vi "CheckShot2Invader_new.vi"(6 "IntensityArray_IN":u8[][](array[numeric]), 7 "InvaderPosArray_IN":T1, 11 "ShotArray_IN":T3[](array[typedef])) -> (3 "ShotArray_OUT":T3[](array[typedef]), 4 "IntensityArray_OUT":u8[][](array[numeric]), 5 "InvaderPosArray_OUT":T1)   [LabVIEW 2022 SP3]
uses:
  InvaderPositionArray.ctl
  move_dir_lr.ctl
  ShotCluster.ctl
  move_dir_ud.ctl
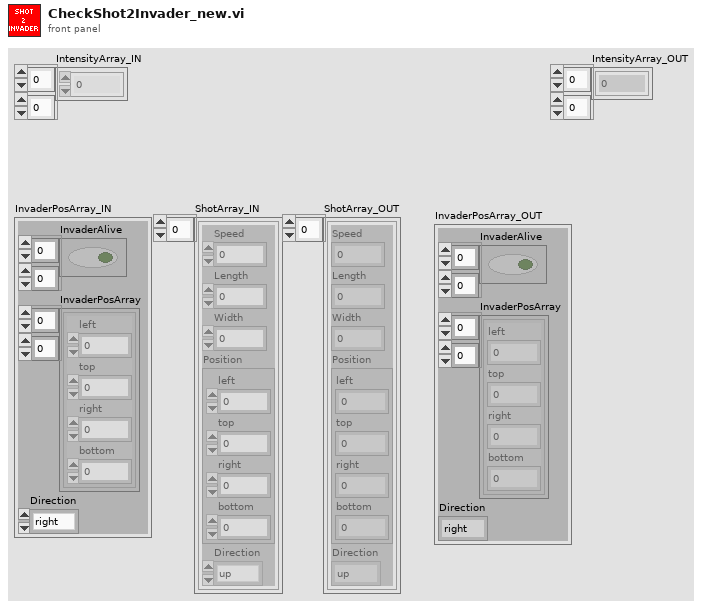
[diagram p1: front panel]
types:
  T1 = typedef "InvaderPositionArray.ctl" = cluster{"InvaderAlive":bool[][], "InvaderPosArray":cluster{"left":i16, "top":i16, "right":i16, "bottom":i16}[][], "Direction":T2}
  T2 = typedef "move_dir_lr.ctl" = enum16{"right", "left"}
  T3 = typedef "ShotCluster.ctl" = cluster{"Speed":u32, "Length":u32, "Width":u32, "Position":cluster{"left":i16, "top":i16, "right":i16, "bottom":i16}, "Direction":T4}
  T4 = typedef "move_dir_ud.ctl" = enum16{"up", "down"}
  T5 = cluster{"left":i16, "top":i16, "right":i16, "bottom":i16}[][]
  T6 = cluster{"left":i16, "top":i16, "right":i16, "bottom":i16}
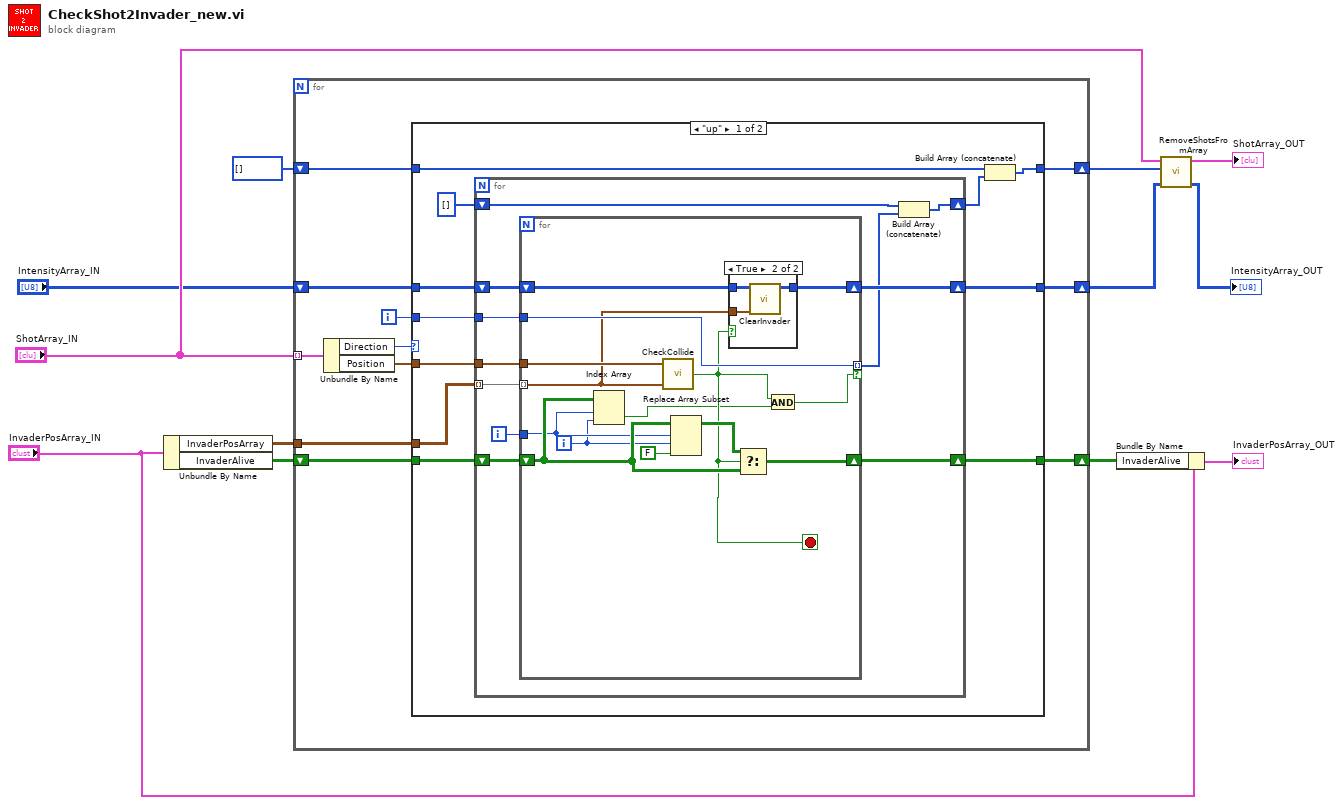
[diagram p0: block diagram]
diagram:
  n1 = Unbundle By Name("InvaderPosArray_IN") -> ("InvaderPosArray"=w1:T5, "InvaderAlive"=w12:bool[][])
  n2 = for {
    tunnel: "ShotArray_IN" -> [w23] mode=indexing
    shift-right: [w19] -> w11
    shift-left: w12 -> [w21]
    shift-right: [w16] -> w5
    shift-left: i32[] [] -> [w17]
    shift-right: [w14] -> w4
    shift-left: "IntensityArray_IN" -> [w15]
    tunnel: w1 -> [w13]
    i -> [w18]
    n3 = Unbundle By Name(w23) -> ("Direction"=w22:T4, "Position"=w20:T6)
    n4 = case shown="\"up\"" w22 {
      tunnel: w21 -> [w33 w66]
      tunnel: w20 -> [w34 _]
      tunnel: [w32 w66] -> w19
      tunnel: w18 -> [w31 _]
      tunnel: w17 -> [w30 w65]
      tunnel: [w28 w65] -> w16
      tunnel: w15 -> [w27 w64]
      tunnel: [w26 w64] -> w14
      tunnel: w13 -> [w25 _]
      frame "up" {
        n5 = for {
          tunnel: w34 -> [w45]
          tunnel: w31 -> [w42]
          tunnel: w25 -> [w39] mode=indexing
          shift-right: [w40] -> w26
          shift-left: w27 -> [w41]
          shift-right: [w38] -> w29
          shift-left: i32[] [] -> [w37]
          shift-right: [w43] -> w32
          shift-left: w33 -> [w44]
          i -> [w35]
          n6 = for {
            tunnel: w45 -> [w59]
            shift-right: [w58] -> w43
            shift-left: w44 -> [w51]
            tunnel: w42 -> [w57]
            tunnel: [w57] -> w36 mode=indexing if=w46
            shift-right: [w55] -> w40
            shift-left: w41 -> [w56]
            tunnel: w39 -> [w54] mode=indexing
            tunnel: w35 -> [w50]
            i -> [w49]
            stop <- w48 stop-if-true
            n7 = Index Array(array=w51, index (row)=w50, index (col)=w49) -> (element=w47:bool)
            n8 = call "CheckCollide.vi"("Rectangle2"=w54, "Rectangle1"=w59) -> ("Collide"=w48:bool)  [unwired: 3 in]
            n9 = Replace Array Subset(array=w51, new element=FALSE, index (row)=w50, index (col)=w49) -> (w52:bool[][])
            n10 = case shown="True" w48 {
              tunnel: w56 -> [w60 w63]
              tunnel: [w60 w62] -> w55
              tunnel: w54 -> [_ w61]
              frame False {
              }
              frame True {
                n11 = call "ClearInvader.vi"("InvaderPosition"=w61, "IntensityArray_IN"=w63) -> ("IntensityArray_OUT"=w62:u8[][])  [unwired: 9 in]
              }
            }
            n12 = Select(t=w52, s=w48, f=w51) -> (s? t:f=w58:bool[][])
            n13 = And(x=w48, y=w47) -> (x .and. y?=w46:bool)
          }
          n14 = Build Array (concatenate)(w37, w36) -> (w38:i32[])
        }
        n15 = Build Array (concatenate)(w30, w29) -> (w28:i32[])
      }
      frame "down" {
      }
    }
  }
  n16 = Bundle By Name(cluster="InvaderPosArray_IN", "InvaderAlive"=w11) -> (→"InvaderPosArray_OUT":T1)
  n17 = call "RemoveShotsFromArray.vi"("IntensityArray_IN"=w4, "Indexes"=w5, "ShotArray_IN"="ShotArray_IN") -> ("IntensityArray_OUT"=→"IntensityArray_OUT":u8[][], "ShotArray_OUT"=→"ShotArray_OUT":T3[])  [unwired: 7 in]
